vi "PV ActiveLine - OffsetCorrection (TPG361).vi"(7 "W/R":bool, 8 "Fehler (Eingang)":errorcluster, 10 "Sensor 1 Set":i8(ring) caption="Sensor 1 Set 2" items=["deactivate", "activate", "set offset and activate", "equalize to zero"], 11 "Referenz in":refnum<visa-resource-name>) -> (0 "Cluster (Ausgang)":errorcluster, 2 "Sensor 1 Get":i8(ring) caption="Sensor 1 Set 2" items=["deactivate", "activate", "set offset and activate", "equalize to zero"], 3 "Referenz out":refnum<visa-resource-name>)   [LabVIEW 2013, in "PV ActiveLine.lvlib"]
doc: "OFC - Offset Correction (Linear Gauges)\n\nTransmit: OFC [,a]\nReceive: a\n\nOffset correction gauge 1,\na =\n0 –> Off (default)\n1 –> On\n2 –> Determine offset value and activate offset correction\n3 –> Adjust the zero of linear gauge"
uses:
  <instrlib>/PV ActiveLine/PV ActiveLine.lvlib
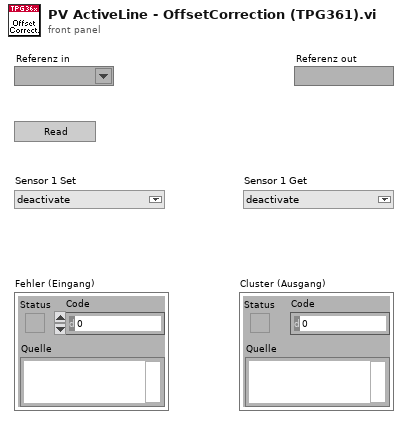
[diagram p1: front panel]
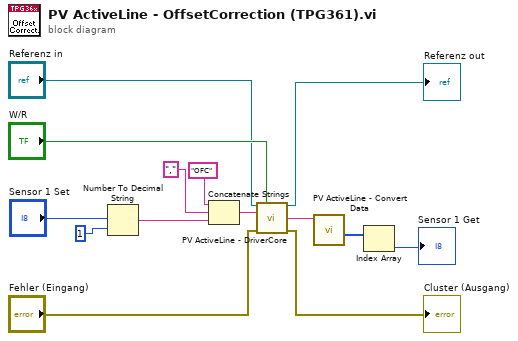
[diagram p0: block diagram]
diagram:
  n1 = Number To Decimal String(number="Sensor 1 Set", width (-)=i16 1) -> (decimal integer string=w3:string)
  n2 = Concatenate Strings("OFC", "," ("Command"), w3) -> (w12:string)
  n3 = call <instrlib>:"PV ActiveLine - DriverCore.vi"("Referenz in"="Referenz in", "Write/Read"="W/R", "Command"=w12, "Fehler (Eingang)"="Fehler (Eingang)") -> ("Referenz out"=→"Referenz out":refnum<visa-resource-name>, "String Out"=w7:string, "Cluster (Ausgang)"=→"Cluster (Ausgang)":errorcluster)  [unwired: 9 in]
  n4 = call <instrlib>:"PV ActiveLine - Convert Data.vi"("String in"=w7) -> ("Integer Out"=w6:i32[])  [unwired: 7 in, 3 out]
  n5 = Index Array(array=w6) -> (element=→"Sensor 1 Get":i32)  [unwired: 1 in]
